vi "Get Size (single).vi"(8 "error in (no error)":errorcluster, 11 "XY-data":cluster{"X-array":dbl[], "Y-array":dbl[]}) -> (0 "error out":errorcluster, 1 "X size":i32, 2 "Y size":i32, 3 "XY-data out":cluster{"X-array":dbl[], "Y-array":dbl[]})   [LabVIEW 2019, in "xy_utilities.lvlib"]
doc: "Get size of X and Y arrays."
uses:
  xy_utilities.lvlib
  Get X and Y (single).vi
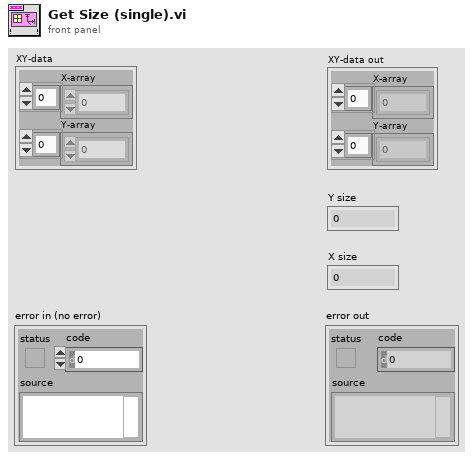
[diagram p1: front panel]
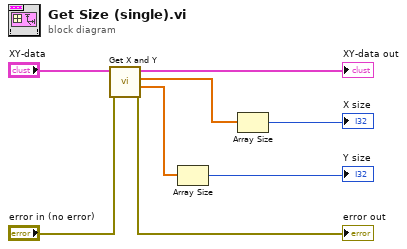
[diagram p0: block diagram]
diagram:
  n1 = call-poly "Get X and Y.vi"("error in (no error)"="error in (no error)", "XY-data"="XY-data") -> ("error out"=→"error out":errorcluster, "Y-array"=w3:dbl[], "X-array"=w1:dbl[], "XY-data out"=→"XY-data out":cluster{"X-array":dbl[], "Y-array":dbl[]})  [unwired: 6 in]
  n2 = Array Size(array=w3) -> (size(s)=→"Y size":i32)
  n3 = Array Size(array=w1) -> (size(s)=→"X size":i32)
